vi "ziExample-UHFLI-ConnectDevice.vi"() -> ()   [LabVIEW 2009]
doc: "Control a Zurich instrument device via the LabOne Labview API. \nRequirements: Zurich Instruments UHFLI \nThis example VI connects and disconnects UHF instruments to a data server using different interfaces.\n\n© Zurich Instruments AG, www.zhinst.com"
uses:
  <instrlib>/Zurich Instruments LabOne/Public/Configure/ziGetValueString.vi
  <vilib>/Utility/error.llb/DialogType.ctl
  <instrlib>/Zurich Instruments LabOne/Zurich Instruments LabOne.lvlib
panel:
  in  "Address":string="localhost:8004"
  in  "Selected Device":i32(listbox)
  in  "Device Interface":string(combo)
  in  "Interface Params (\"\")":string
  in  "DisConnectDevice":bool
  in  "ConnectDevice":bool
  in  "Available Devices":i32(listbox)
  in  "Update":bool
  in  "Stop":bool
  out "Error Out":errorcluster
  # "Tested Instruments:\n- UHFLI"
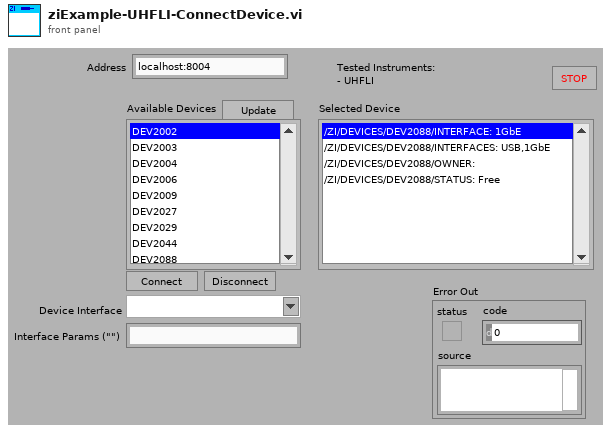
[diagram p1: front panel]
types:
  T1 = typedef "Zurich Instruments LabOne.lvlib/ziTypeHandle.ctl" = cluster{"handleValid":bool, "Conn":u64, "Path Prefix":string, "Handle":u64, "Connected":bool, "Clockbase(s)":dbl}
  T2 = typedef "DialogType.ctl" = u16
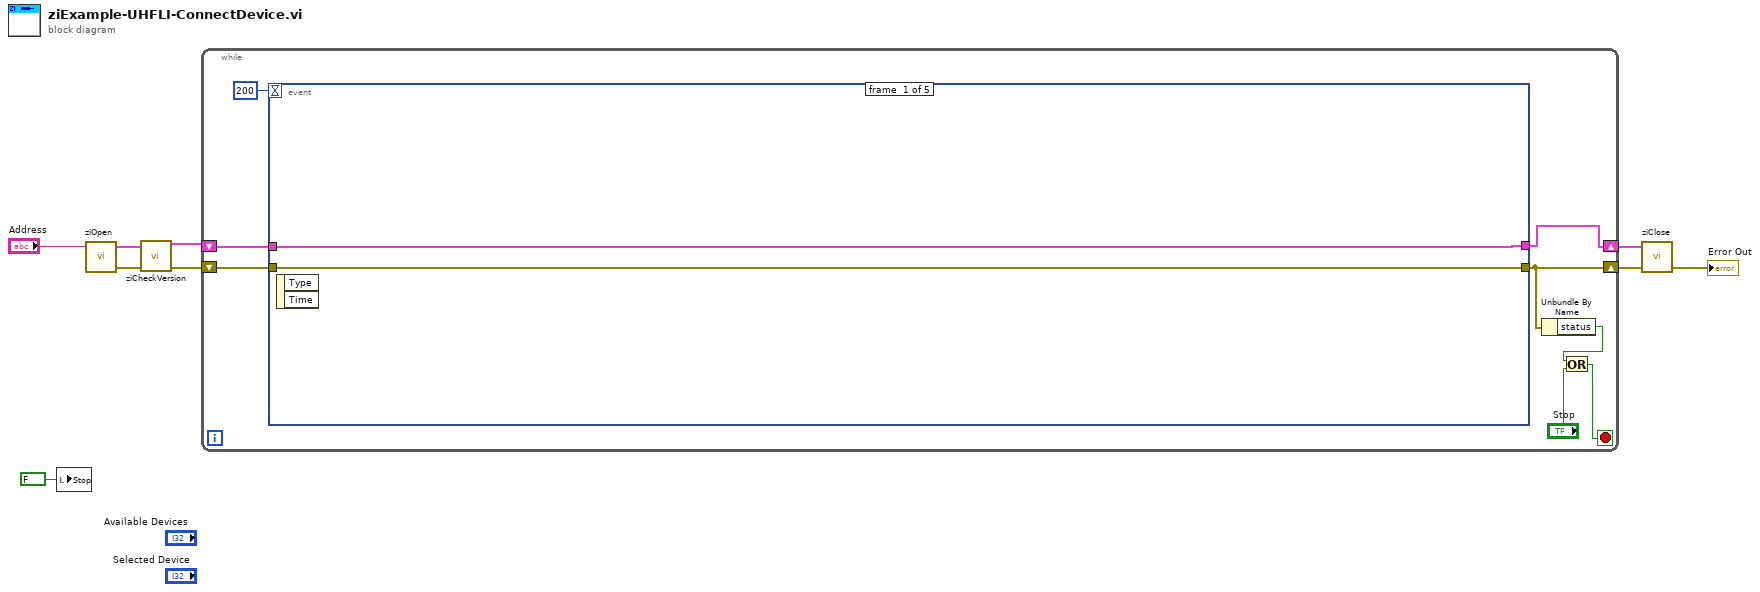
[diagram p0: block diagram]
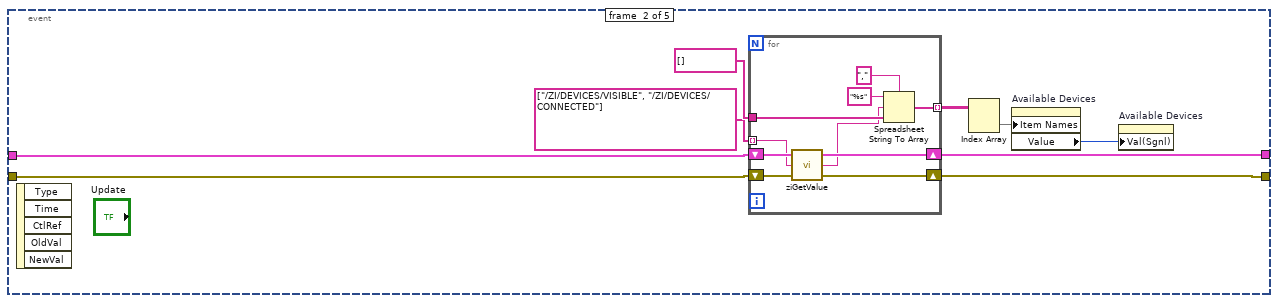
[diagram p2: hidden frame]
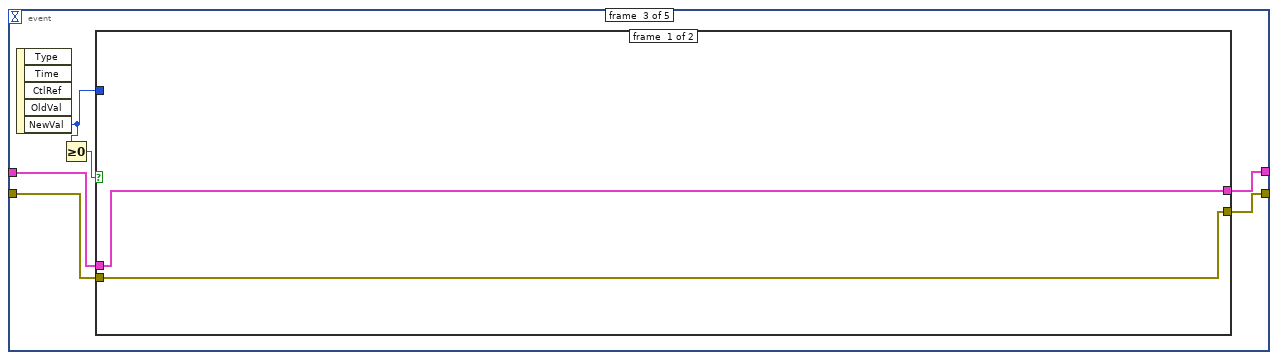
[diagram p3: hidden frame]
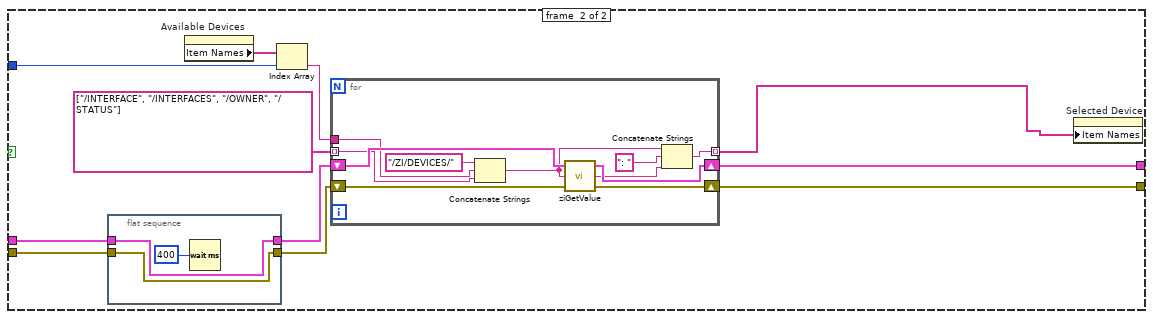
[diagram p4: hidden frame]
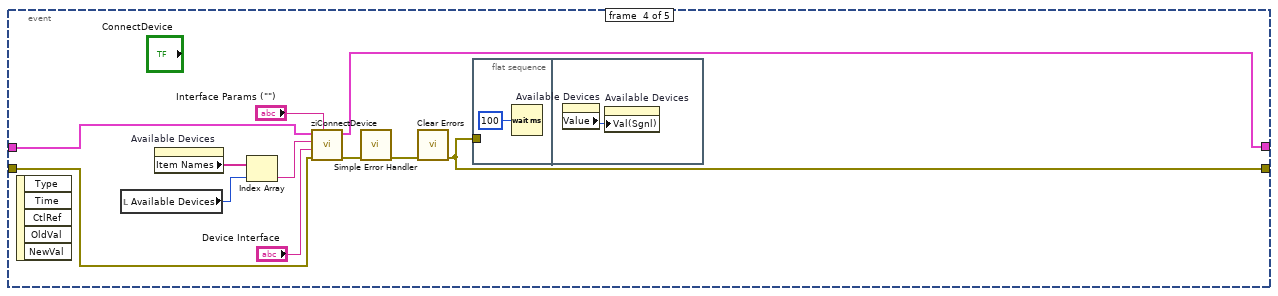
[diagram p5: hidden frame]
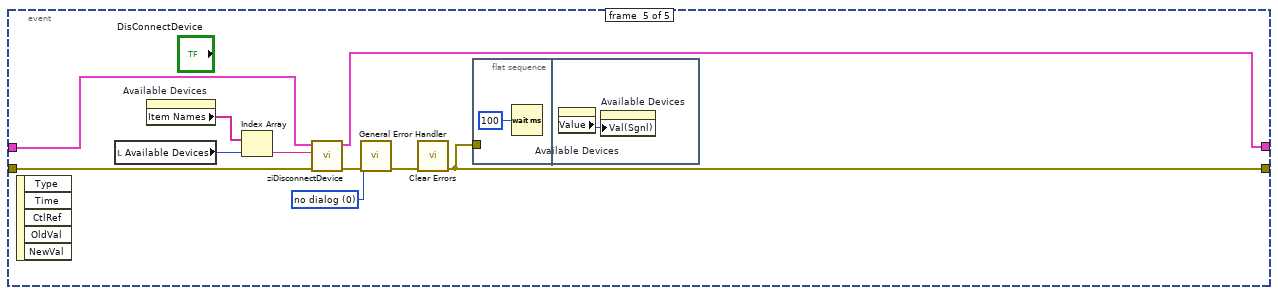
[diagram p6: hidden frame]
diagram:
  n1 = local write "Stop"(FALSE ("Stop")) -> ()
  n2 = call <instrlib>:"ziOpen.vi"("Address"="Address") -> ("Error Out"=w4:errorcluster, "HandleOut"=w5:T1)  [unwired: 1 in, 3 out]
  n3 = call <instrlib>:"ziCheckVersion.vi"("Handle In"=w5, "Error In"=w4) -> ("Handle Out"=w3:T1, "Error Out"=w2:errorcluster)  [unwired: 11 in, 1 out]
  n4 = while {
    shift-right: [w15] -> w9
    shift-left: w3 -> [w17]
    shift-right: [w10] -> w8
    shift-left: w2 -> [w16]
    stop <- w13 stop-if-true
    n5 = event shown="[2] \"Available Devices\": Value Change" {
      selector: _ -> [_ _ _ _ _]
      dyn-events: _ -> [_ _ _ _ _]
      timeout: 200 -> [_ _ _ _ _]
      tunnel: w17 -> [w19 w21 w43 w81 w93]
      tunnel: w16 -> [w18 w20 w44 w80 w92]
      tunnel: [w19 w26 w42 w82 w94] -> w15
      tunnel: [w18 w28 w41 w72 w86] -> w10
      event #0 {
        n6 = event-data() -> ()  [unwired: 1 in, 2 out]
      }
      event #1 {
        n7 = event-data() -> ()  [unwired: 1 in, 5 out]
        n8 = for {
          shift-right: [w35] -> w26
          shift-left: w21 -> [w36]
          shift-right: [w37] -> w28
          shift-left: w20 -> [w38]
          tunnel: string[] [] ("array") -> [w32]
          tunnel: [w31] -> w23 mode=indexing
          tunnel: string[] ["/ZI/DEVICES/VISIBLE", "/ZI/DEVICES/CONNECTED"] -> [w29] mode=indexing
          n9 = call-poly <instrlib>:"ziGetValue.vi"("error in"=w38, "Path"=w29, "Handle In"=w36) -> ("error out"=w37:errorcluster, "Value"=w30:string, "Handle Out"=w35:T1)
          n10 = Spreadsheet String To Array(delimiter (Tab)=",", format string="%s", spreadsheet string=w30, array type (2D Dbl)=w32) -> (array=w31:string[])
        }
        n11 = Index Array(array=w23) -> (element=w24:string[])  [unwired: 2 in]
        n12 = property on="Available Devices" class="LstBox (strict)"("Item Names"=w24) -> ("Value"=w22:i32)  [unwired: 2 in, 2 out]
        n13 = property on="Available Devices" class="LstBox (strict)"("Val(Sgnl)"=w22) -> ()  [unwired: 2 in, 2 out]
      }
      event #2 {
        n14 = event-data() -> ("NewVal"=w39:i32)  [unwired: 1 in, 4 out]
        n15 = Greater Or Equal To 0?(x=w39) -> (x >= 0?=w40:bool)
        n16 = case shown="True" w40 {
          tunnel: w39 -> [_ w53]
          tunnel: w44 -> [w45 w52]
          tunnel: w43 -> [w46 w51]
          tunnel: [w46 w49] -> w42
          tunnel: [w45 w48] -> w41
          frame #0 {
          }
          frame #1 {
            n17 = flat-sequence {
              tunnel: w51 -> [w59]
              tunnel: w52 -> [w60]
              tunnel: [w60] -> w56
              tunnel: [w59] -> w55
              frame #0 {
                n18 = Wait (ms)(milliseconds to wait=u32 400) -> ()  [unwired: 1 out]
              }
            }
            n19 = property on="Available Devices" class="LstBox (strict)"() -> ("Item Names"=w54:string[])  [unwired: 2 in, 2 out]
            n20 = Index Array(array=w54, index=w53) -> (element=w50:string)
            n21 = for {
              tunnel: string[] ["/INTERFACE", "/INTERFACES", "/OWNER", "/STATUS"] -> [w64] mode=indexing
              shift-right: [w70] -> w49
              shift-left: w55 -> [w71]
              tunnel: [w69] -> w47 mode=indexing
              shift-right: [w67] -> w48
              shift-left: w56 -> [w68]
              tunnel: w50 -> [w62]
              n22 = Concatenate Strings("/ZI/DEVICES/" ("string"), w62, w64) -> (w61:string)
              n23 = call-poly <instrlib>:"ziGetValue.vi"("error in"=w68, "Path"=w61, "Handle In"=w71) -> ("error out"=w67:errorcluster, "Value"=w66:string, "Handle Out"=w70:T1)
              n24 = Concatenate Strings(w61, ": " ("string"), w66) -> (w69:string)
            }
            n25 = property on="Selected Device" class="LstBox (strict)"("Item Names"=w47) -> ()  [unwired: 2 in, 2 out]
          }
        }
      }
      event #3 {
        n26 = event-data() -> ()  [unwired: 1 in, 5 out]
        n27 = local read "Available Devices"() -> (w75:i32)
        n28 = property on="Available Devices" class="LstBox (strict)"() -> ("Item Names"=w77:string[])  [unwired: 2 in, 2 out]
        n29 = Index Array(array=w77, index=w75) -> (element=w76:string)
        n30 = call <instrlib>:"ziConnectDevice.vi"("Device Interface Params (\"\")"="Interface Params (\"\")", "Error In"=w80, "Device Interface"="Device Interface", "Device Serial"=w76, "Handle In"=w81) -> ("Error Out"=w79:errorcluster, "Handle Out"=w82:T1)  [unwired: 5 in]
        n31 = call <vilib>:"Simple Error Handler.vi"("error in (no error)"=w79) -> ("error out"=w73:errorcluster)  [unwired: 4 in, 4 out]
        n32 = call <vilib>:"Clear Errors.vi"("error in (no error)"=w73) -> ("error out"=w72:errorcluster)  [unwired: 6 in]
        n33 = flat-sequence {
          tunnel: w72 -> [_]
          frame #0 {
            n34 = Wait (ms)(milliseconds to wait=u32 100) -> ()  [unwired: 1 out]
          }
          frame #1 {
            n35 = property on="Available Devices" class="LstBox (strict)"() -> ("Value"=w84:i32)  [unwired: 2 in, 2 out]
            n36 = property on="Available Devices" class="LstBox (strict)"("Val(Sgnl)"=w84) -> ()  [unwired: 2 in, 2 out]
          }
        }
      }
      event #4 {
        w85 = T2 0 items=["no dialog", "OK message", "continue or stop message", "OK message + warnings", "continue/stop + warnings"] ("type of dialog (OK msg:1)")
        n37 = event-data() -> ()  [unwired: 1 in, 5 out]
        n38 = local read "Available Devices"() -> (w89:i32)
        n39 = property on="Available Devices" class="LstBox (strict)"() -> ("Item Names"=w91:string[])  [unwired: 2 in, 2 out]
        n40 = Index Array(array=w91, index=w89) -> (element=w90:string)
        n41 = call <instrlib>:"ziDisconnectDevice.vi"("Error In"=w92, "Device Serial"=w90, "Handle In"=w93) -> ("Error Out"=w87:errorcluster, "Handle Out"=w94:T1)  [unwired: 7 in]
        n42 = call <vilib>:"General Error Handler.vi"("type of dialog (OK msg:1)"=w85, "error in (no error)"=w87) -> ("error out"=w88:errorcluster)  [unwired: 9 in, 4 out]
        n43 = call <vilib>:"Clear Errors.vi"("error in (no error)"=w88) -> ("error out"=w86:errorcluster)  [unwired: 6 in]
        n44 = flat-sequence {
          tunnel: w86 -> [_]
          frame #0 {
            n45 = Wait (ms)(milliseconds to wait=u32 100) -> ()  [unwired: 1 out]
          }
          frame #1 {
            n46 = property on="Available Devices" class="LstBox (strict)"() -> ("Value"=w96:i32)  [unwired: 2 in, 2 out]
            n47 = property on="Available Devices" class="LstBox (strict)"("Val(Sgnl)"=w96) -> ()  [unwired: 2 in, 2 out]
          }
        }
      }
    }
    n48 = Unbundle By Name(w10) -> ("status"=w11:bool)
    n49 = Or(x=w11, y="Stop") -> (x .or. y?=w13:bool)
  }
  n50 = call <instrlib>:"ziClose.vi"("Error In"=w8, "Handle In"=w9) -> ("Error Out"=→"Error Out":errorcluster)  [unwired: 3 out]
